vi "GameEl_Init.vi"(8 "Error In":errorcluster, 11 "object in":refnum<class "GameEl.lvclass">) -> (0 "Error Out":errorcluster, 3 "object out":refnum<class "GameEl.lvclass">)   [LabVIEW 2021, in "GameEl.lvclass"]
uses:
  GameEl.lvclass
  GameEl.lvclass/GameEl.ctl
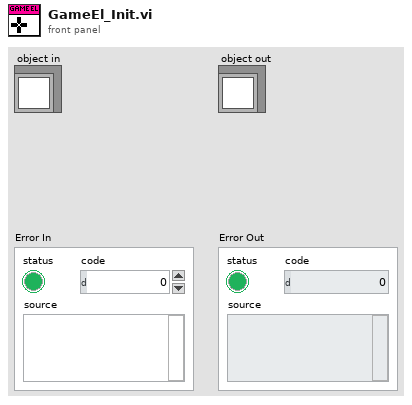
[diagram p1: front panel]
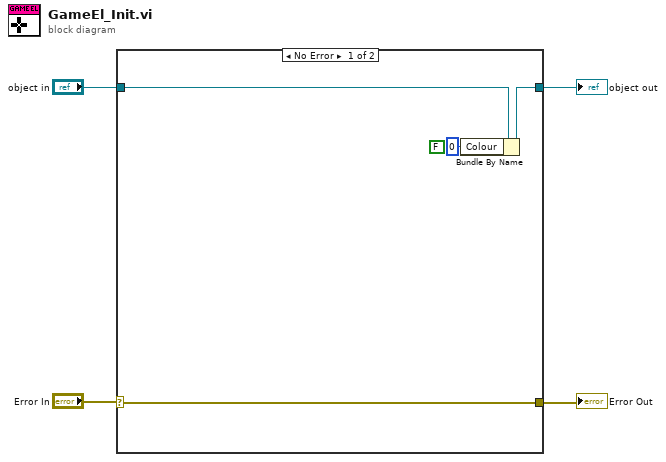
[diagram p0: block diagram]
diagram:
  n1 = case shown="No Error" "Error In" {
    selector: "Error In" -> [w6 w9]
    tunnel: "object in" -> [w8 w10]
    tunnel: [w7 w10] -> w3
    tunnel: [w6 w9] -> w1
    frame No Error {
      (unwired) FALSE ("None")
      n2 = Bundle By Name(cluster=w8, "Colour"=u32 0) -> (w7:refnum<class "GameEl.lvclass">)
    }
    frame Error {
    }
  }
  "object out" <- w3
  "Error Out" <- w1
